vi "programa11.vi"() -> ()   [LabVIEW 2011]
uses:
  <vilib>/express/express arith-compare/Formula/XNode/ExpressFormulaBlockNode.xnode
panel:
  out "Menor":dbl
  out "Mayor":dbl
  out "Promedio":dbl
  out "Contador":dbl
  out "NumeroPar":dbl
  # "Elaborar un programa donde  se generen y presenten 5 \nnumeros pares. obtener el promedio , el numero mayor y menor"
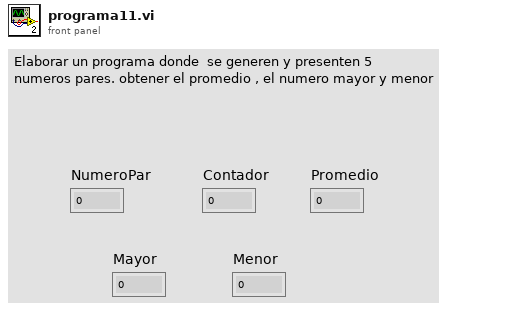
[diagram p1: front panel]
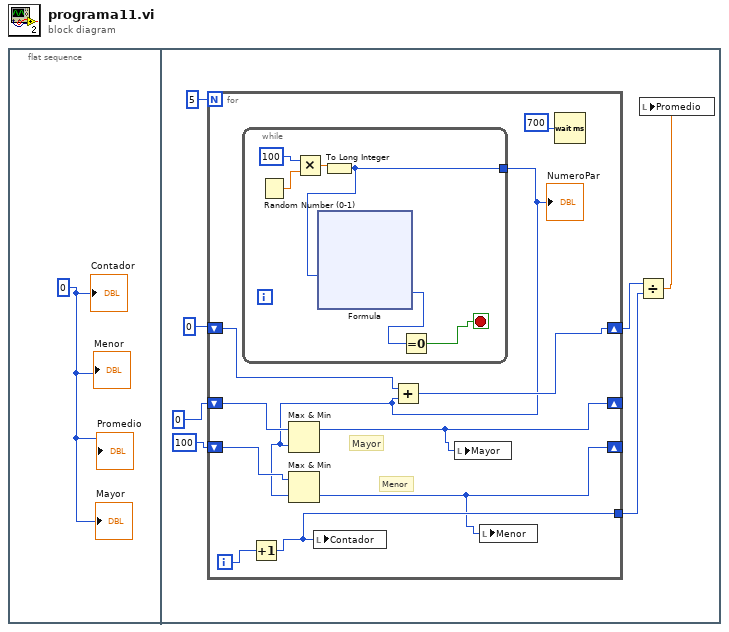
[diagram p0: block diagram]
diagram:
  n1 = flat-sequence {
    frame #0 {
      w1 = 0
      "Contador" <- w1
      "Menor" <- w1
      "Promedio" <- w1
      "Mayor" <- w1
    }
    frame #1 {
      n2 = for {
        N: 5 -> [_]
        shift-right: [w16] -> w6
        shift-left: 0 -> [w17]
        tunnel: [w15] -> w5
        shift-right: [w11] -> _
        shift-left: 0 -> [w14]
        shift-right: [w10] -> _
        shift-left: 100 -> [w13]
        i -> [w18]
        # "Menor"
        # "Mayor"
        n3 = while {
          tunnel: [w19] -> w12
          stop <- w20 stop-if-true
          n4 = Random Number (0-1)() -> (number: 0 to 1=w23:dbl)
          n5 = Multiply(x=100, y=w23) -> (x*y=w22:dbl)
          n6 = To Long Integer(number=w22) -> (32bit integer=w19:i32)
          n7 = xnode "Formula"("X1"=w19) -> ("Result"=w21:i32)  [unwired: 1 in, 1 out]
          n8 = Equal To 0?(x=w21) -> (x = 0?=w20:bool)
        }
        "NumeroPar" <- w12
        n9 = Increment(x=w18) -> (x+1=w15:i32)
        n10 = Max & Min(x=w14, y=w12) -> (max(x,y)=w11:i32)  [unwired: 1 out]
        n11 = Max & Min(x=w13, y=w12) -> (min(x,y)=w10:i32)  [unwired: 1 out]
        n12 = local write "Contador"(w15) -> ()
        n13 = Add(x=w17, y=w12) -> (x+y=w16:i32)
        n14 = local write "Mayor"(w11) -> ()
        n15 = local write "Menor"(w10) -> ()
        n16 = Wait (ms)(milliseconds to wait=700) -> ()  [unwired: 1 out]
      }
      n17 = Divide(x=w6, y=w5) -> (x/y=w4:dbl)
      n18 = local write "Promedio"(w4) -> ()
    }
  }
